vi "Add Table Columns.vi"(8 "error in (no error)":errorcluster caption="错误输入（无错误）", 9 "DataColunm Types":variant[](array[variant]), 10 "DataColumn Names":string[](array[string]), 11 "DataTable 输入":refnum<class "DataTable.lvclass"> caption="DNL_LabVIEW Object in") -> (0 "error out":errorcluster caption="错误输出", 3 "DataTable 输出":refnum<class "DataTable.lvclass"> caption="DNL_LabVIEW Object out")   [LabVIEW 2012, in "Data Grid VIEW.lvlib" / "DataTable.lvclass"]
uses:
  DataTable.lvclass
  DataTable.lvclass/DataTable.ctl
  Data Column/Data Column.lvclass/Data Column.ctl
  System.Data
  Data Column/Data Column.lvclass
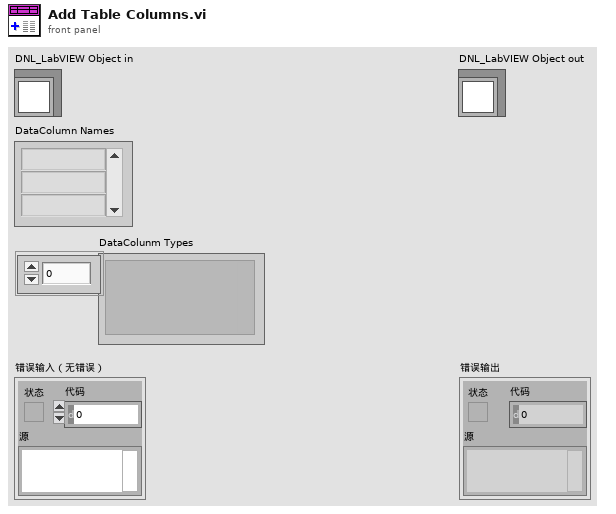
[diagram p1: front panel]
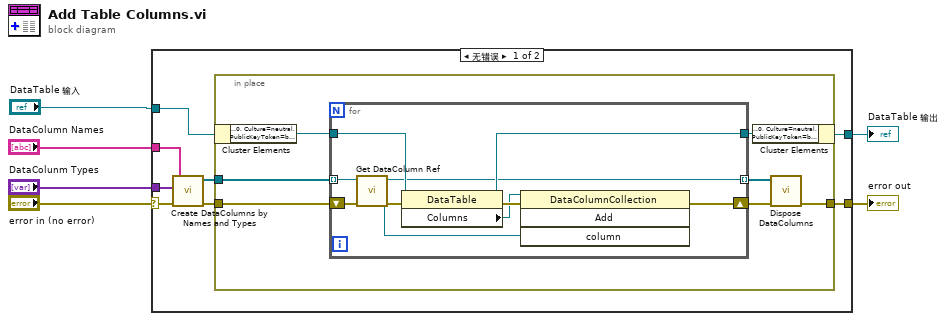
[diagram p0: block diagram]
diagram:
  n1 = case shown="无错误" "error in (no error)" {
    selector: "error in (no error)" -> [w12 w32]
    tunnel: [w8 w33] -> w4
    tunnel: "DataTable 输入" -> [w11 w33]
    tunnel: "DataColumn Names" -> [w14 _]
    tunnel: "DataColunm Types" -> [w13 _]
    tunnel: [w7 w32] -> w1
    frame No Error {
      n2 = call "Create DataColumns by Names and Types.vi"("error in (no error)"=w12, "DataColunm Types"=w13, "DataColumn Names"=w14) -> ("error out"=w9:errorcluster, "DataColumns"=w10:refnum<class "Data Column.lvclass">[])  [unwired: 7 in]
      n3 = in-place {
        in-place-border: w10 -> [w19]
        in-place-border: w9 -> [w20]
        in-place-border: [w16] -> w7
        n4 = in-place-cluster #1(w11) -> ("DataTable"=w21:refnum<k24>)
        n5 = for {
          tunnel: w21 -> [w30]
          shift-right: [w23] -> w17
          shift-left: w20 -> [w27]
          tunnel: w19 -> [w28] mode=indexing
          tunnel: [w24] -> w18
          tunnel: [w22] -> w15 mode=indexing
          n6 = call "Get DataColumn Ref.vi"("error in (no error)"=w27, "Data Column输入"=w28) -> ("error out"=w26:errorcluster, "DataColumn"=w25:refnum<k24>, "Data Column输出"=w22:refnum<class "Data Column.lvclass">)  [unwired: 7 in]
          n7 = property class="DataTable"(reference=w30, error in=w26) -> (reference out=w24:refnum<k24>, error out=w31:errorcluster, "Columns"=w29:refnum<k24>)
          n8 = invoke class="DataColumnCollection" method="Add"(reference=w29, error in=w31, "column"=w25) -> (error out=w23:errorcluster)  [unwired: 1 in, 3 out]
        }
        n9 = in-place-cluster #1("DataTable"=w18) -> (w8:refnum<class "DataTable.lvclass">)
        n10 = call "Dispose DataColumns.vi"("error in (no error)"=w17, "DataColumns"=w15) -> ("error out"=w16:errorcluster)  [unwired: 9 in]
      }
    }
    frame Error {
    }
  }
  "error out" <- w1
  "DataTable 输出" <- w4
